vi "Main_SubVI_Sort Comment (Read).vi"(8 "Error In":errorcluster, 9 "Number":i32, 10 "Register  Address":i32, 11 "Axis Number":T1=1 items=["X"=1, "Y"=2, "Z"=3, "Rotation"=4]) -> (0 "Error Out":errorcluster, 3 "Command":string)   [LabVIEW 2015]
uses:
  Control/Control_Axis Number.ctl
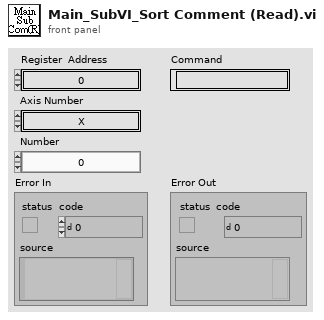
[diagram p1: front panel]
types:
  T1 = typedef "Control_Axis Number.ctl" = u16
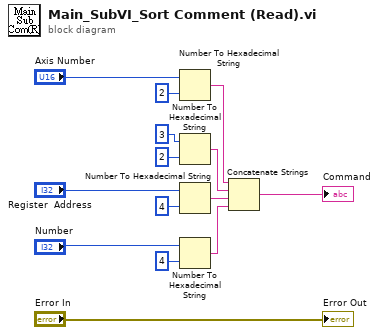
[diagram p0: block diagram]
diagram:
  n1 = Number To Hexadecimal String(1:i16 2 ("width (-)"), 2:"Axis Number") -> (0:w10:string)
  n2 = Number To Hexadecimal String(1:i16 2 ("width (-)"), 2:3 ("number")) -> (0:w9:string)
  n3 = Number To Hexadecimal String(1:i16 4 ("width (-)"), 2:"Register  Address") -> (0:w8:string)
  n4 = Number To Hexadecimal String(1:i16 4 ("width (-)"), 2:"Number") -> (0:w6:string)
  n5 = Concatenate Strings(w10, w9, w8, w6) -> (→"Command":string)
  "Error Out" <- "Error In"
